vi "OnResize2.vi"(0 "XRef":T9, 1 "Bounds":T7, 2 "Mouse Mods":T5, 3 "State In":T1) -> (14 "Reply":T3, 15 "Fatal Error Out":T2, 16 "State Out":T1)   [LabVIEW 2015, in "Set Object Parameters.xnode"]
uses:
  Set Object Parameters.xnode
  <vilib>/XNodeSupport/XNodeXNodeRef.ctl
  <vilib>/XNodeSupport/XNodeRect32.ctl
  <vilib>/XNodeSupport/XNodeInt.ctl
  <vilib>/XNodeSupport/XNodeMouseMods.ctl
  <vilib>/XNodeSupport/XNodeBool.ctl
  State.ctl
  <vilib>/XNodeSupport/XNodeStringArray.ctl
  <vilib>/XNodeSupport/XNodeString.ctl
  <vilib>/XNodeSupport/XNodeErrorCluster.ctl
  dimensions.vi
  <vilib>/XNodeSupport/NI_XNodeSupport.lvlib
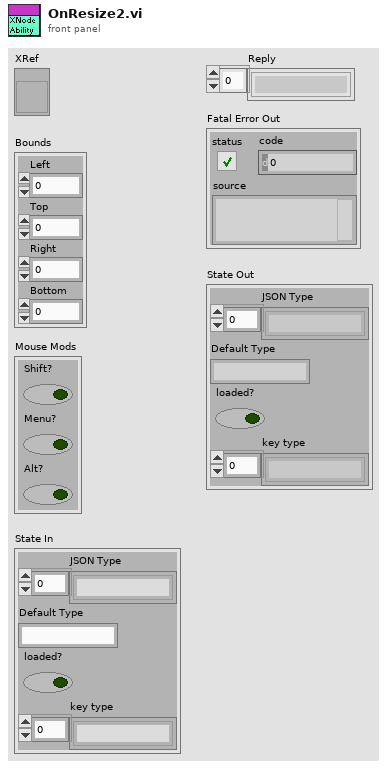
[diagram p1: front panel]
types:
  T1 = typedef "Set Object Parameters.xnode/State.ctl" = cluster{"JSON Type":string[], "Default Type":string, "loaded?":bool, "key type":string[]}
  T2 = typedef "NI_XNodeSupport.lvlib/XNodeErrorCluster.ctl" = errorcluster
  T3 = typedef "NI_XNodeSupport.lvlib/XNodeStringArray.ctl" = T4[]
  T4 = typedef "NI_XNodeSupport.lvlib/XNodeString.ctl" = string
  T5 = typedef "NI_XNodeSupport.lvlib/XNodeMouseMods.ctl" = cluster{"Shift?":T6, "Menu?":T6, "Alt?":T6}
  T6 = typedef "NI_XNodeSupport.lvlib/XNodeBool.ctl" = bool
  T7 = typedef "NI_XNodeSupport.lvlib/XNodeRect32.ctl" = cluster{"Left":T8, "Top":T8, "Right":T8, "Bottom":T8}
  T8 = typedef "NI_XNodeSupport.lvlib/XNodeInt.ctl" = i32
  T9 = typedef "NI_XNodeSupport.lvlib/XNodeXNodeRef.ctl" = refnum<vi>
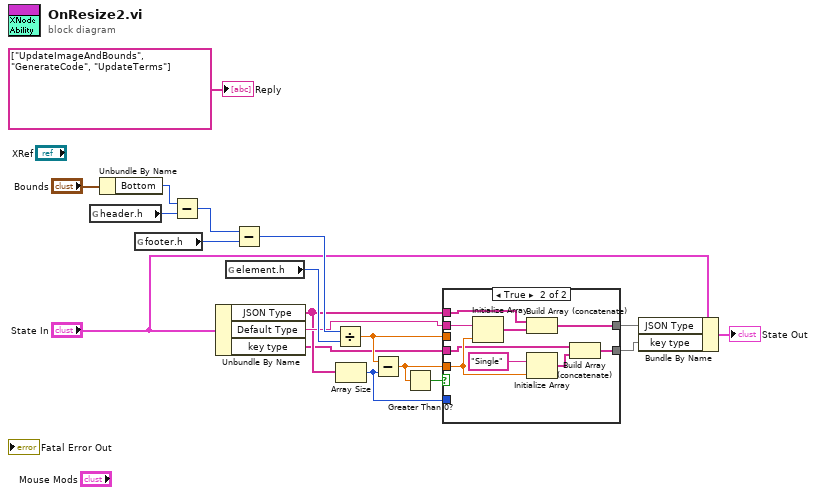
[diagram p0: block diagram]
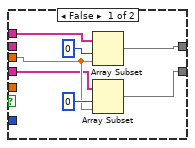
[diagram p2: hidden frame]
diagram:
  n1 = global read "dimensions.vi" "header.h"() -> (w13:i16)
  n2 = Unbundle By Name("Bounds") -> ("Bottom"=w15:T8)
  n3 = global read "dimensions.vi" "footer.h"() -> (w12:i16)
  n4 = Subtract(x=w15, y=w13) -> (x-y=w14:T8)
  n5 = Unbundle By Name("State In") -> ("JSON Type"=w4:string[], "Default Type"=w5:string, "key type"=w2:string[])
  n6 = global read "dimensions.vi" "element.h"() -> (w16:i16)
  n7 = Subtract(x=w14, y=w12) -> (x-y=w11:T8)
  n8 = Divide(x=w11, y=w16) -> (x/y=w6:dbl)
  n9 = Array Size(array=w4) -> (size(s)=w3:i32)
  n10 = Subtract(x=w6, y=w3) -> (x-y=w8:dbl)
  n11 = Greater Than 0?(x=w8) -> (x > 0?=w9:bool)
  n12 = case shown="True" w9 {
    tunnel: w8 -> [_ w30]
    tunnel: w4 -> [w26 w35]
    tunnel: [w25 w33] -> w7
    tunnel: w3 -> [_ _]
    tunnel: w6 -> [w22 _]
    tunnel: w5 -> [_ w32]
    tunnel: w2 -> [w21 w29]
    tunnel: [w20 w27] -> w1
    frame False {
      n13 = Array Subset(array=w26, index=0, length=w22) -> (w25:string[])
      n14 = Array Subset(array=w21, index=0, length=w22) -> (w20:string[])
    }
    frame True {
      n15 = Initialize Array(w32, w30) -> (w34:string[])
      n16 = Build Array (concatenate)(w35, w34) -> (w33:string[])
      n17 = Initialize Array("Single" ("element"), w30) -> (w28:string[])
      n18 = Build Array (concatenate)(w29, w28) -> (w27:string[])
    }
  }
  n19 = Bundle By Name(cluster="State In", "JSON Type"=w7, "key type"=w1) -> (→"State Out":T1)
  "Reply" <- T3 ["UpdateImageAndBounds", "GenerateCode", "UpdateTerms"] ("Reply")
